vi "Panel-FringeProcessor-1.vi"() -> ()   [LabVIEW 2009]
uses:
  <vilib>/Analysis/2dsp.llb/Real FFT.vi
  <vilib>/Analysis/NI_AALPro.lvlib
panel:
  out "Waveform Graph":dbl[](graph)
  in  "stop":bool
  out "Individual Spots":i32[](graph)
  out "Intensity Graph":i32[][](graph)
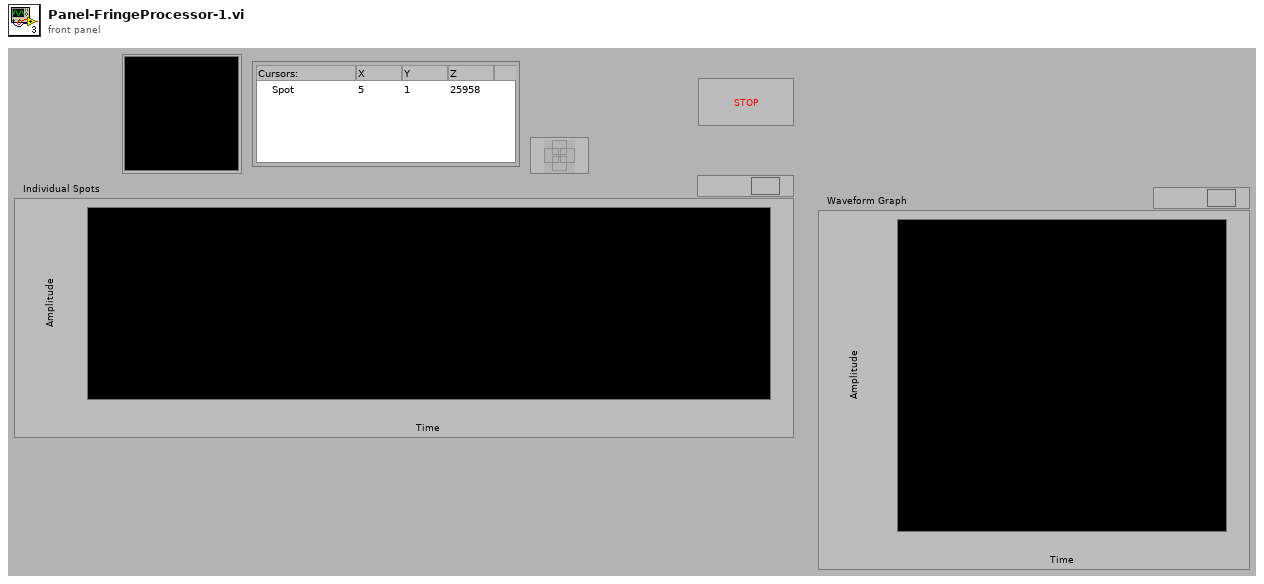
[diagram p1: front panel]
types:
  T1 = typedef "NICMOS.DATA.ctl" = cluster{"DATA":i32[][][], "INDEX":i32}
  T2 = typedef "LVPointDoubleTypeDef.ctl" = cluster{"Cursor X":dbl, "Cursor Y":dbl}
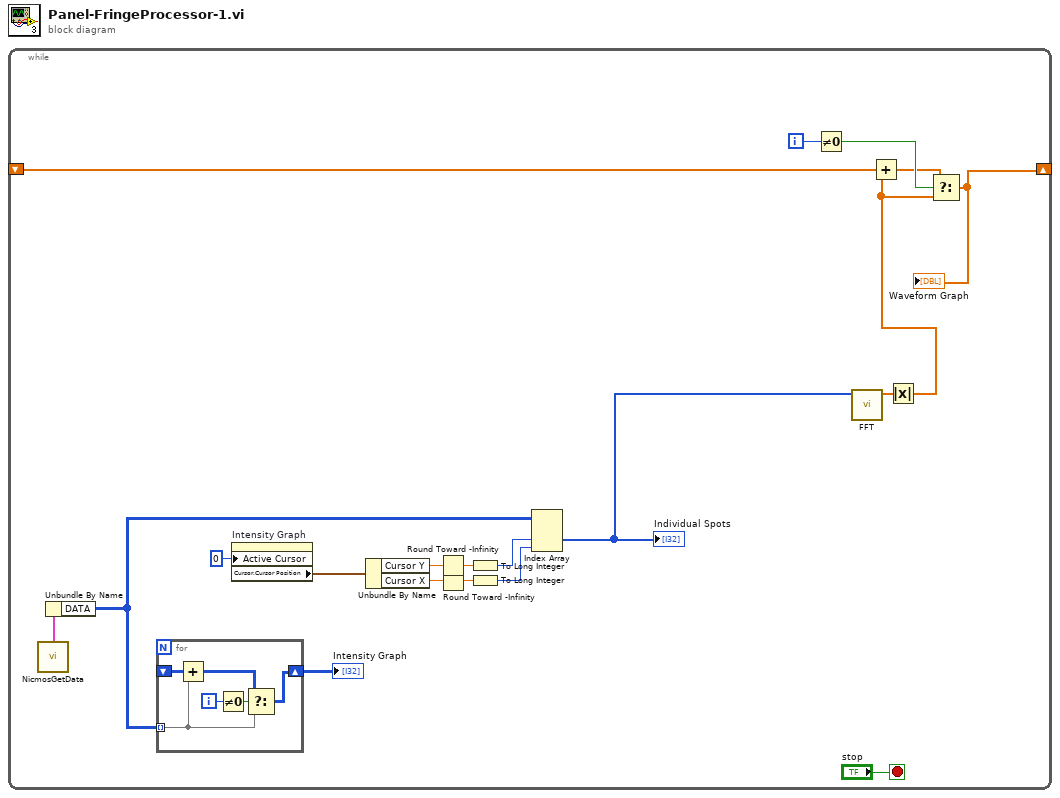
[diagram p0: block diagram]
diagram:
  n1 = while {
    shift-right: [w1] -> _
    shift-left: _ -> [w16]
    i -> [w15]
    stop <- "stop" stop-if-true
    n2 = call "NicmosGetData.vi"() -> ("DATA"=w20:T1)  [unwired: 8 in, 1 out]
    n3 = Unbundle By Name(w20) -> ("DATA"=w18:i32[][][])
    n4 = for {
      tunnel: w18 -> [w22] mode=indexing
      shift-right: [w24] -> w19
      shift-left: _ -> [w23]
      i -> [w26]
      n5 = Add(x=w23, y=w22) -> (x+y=w21:i32[][])
      n6 = Not Equal To 0?(x=w26) -> (x != 0?=w25:bool)
      n7 = Select(t=w21, s=w25, f=w22) -> (s? t:f=w24:i32[][])
    }
    "Intensity Graph" <- w19
    n8 = property on="Intensity Graph" class="IntGraph (strict)"("Active Cursor"=u32 0) -> ("Cursor.Cursor Position"=w5:T2)  [unwired: 2 in, 2 out]
    n9 = Unbundle By Name(w5) -> ("Cursor Y"=w11:dbl, "Cursor X"=w10:dbl)
    n10 = Round Toward -Infinity(1:w11) -> (0:w9:dbl)
    n11 = Round Toward -Infinity(1:w10) -> (0:w8:dbl)
    n12 = To Long Integer(number=w9) -> (32bit integer=w7:i32)
    n13 = To Long Integer(number=w8) -> (32bit integer=w6:i32)
    n14 = Index Array(array=w18, index (dim 1)=w7, index (dim 2)=w6) -> (element=w3:i32[])  [unwired: 1 in]
    "Individual Spots" <- w3
    n15 = Not Equal To 0?(x=w15) -> (x != 0?=w14:bool)
    n16 = call-poly <vilib>:"FFT.vi"("X"=w3) -> ("FFT {X}"=w12:cdb[])  [unwired: 9 in, 1 out]
    n17 = Absolute Value(x=w12) -> (abs(x)=w2:dbl[])
    n18 = Add(x=w16, y=w2) -> (x+y=w13:dbl[])
    n19 = Select(t=w13, s=w14, f=w2) -> (s? t:f=w1:dbl[])
    "Waveform Graph" <- w1
  }
